vi "RC_STM_Client 1.vi"() -> ()   [LabVIEW 2019, in "RemoteControl.STM.lvclass"]
uses:
  RemoteControl.STM.lvclass
  RemoteControl/RemoteControl.lvclass
  <userlib>/_OpenG.lib/numeric/numeric.llb/Random Number Within Range - I32__ogtk.vi
  <userlib>/_OpenG.lib/error/error.llb/Filter Error Codes (Array)__ogtk.vi
  RemoteControl/Typedefs/RC Com Type--enum.ctl
panel:
  in  "Test RC Client":bool
  in  "milliseconds to wait":u32
  out "time (1 message) (ms)":u32
  out "startup time (ms)":u32
  out "messsages/s":dbl
  in  "remote port":u16=6341
  in  "address":string
  out "Data reponse":string
  out "Messages":i32
  in  "Stop":bool
  out "Command reponse":string
  out "Command":string
  out "meta data\n(available commands)":string
  out "error out":errorcluster
  # "CLIENT (API)"
  # "Connection info"
  # "Message Sent"
  # "Message Received"
  # "Metrics"
  # "1"
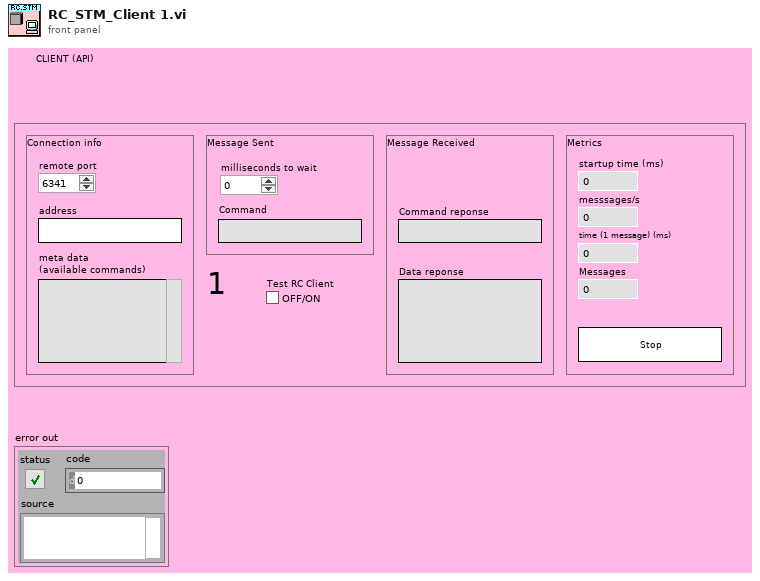
[diagram p1: front panel]
types:
  T1 = typedef "RemoteControl.lvclass/RC Com Type--enum.ctl" = enum16{"RC", "STM", "ZMQ"}
  T2 = typedef "NI STM.lvlib/MetaDataElement.ctl" = string
  T3 = cluster{"Command out":string, "Data out":variant, string}
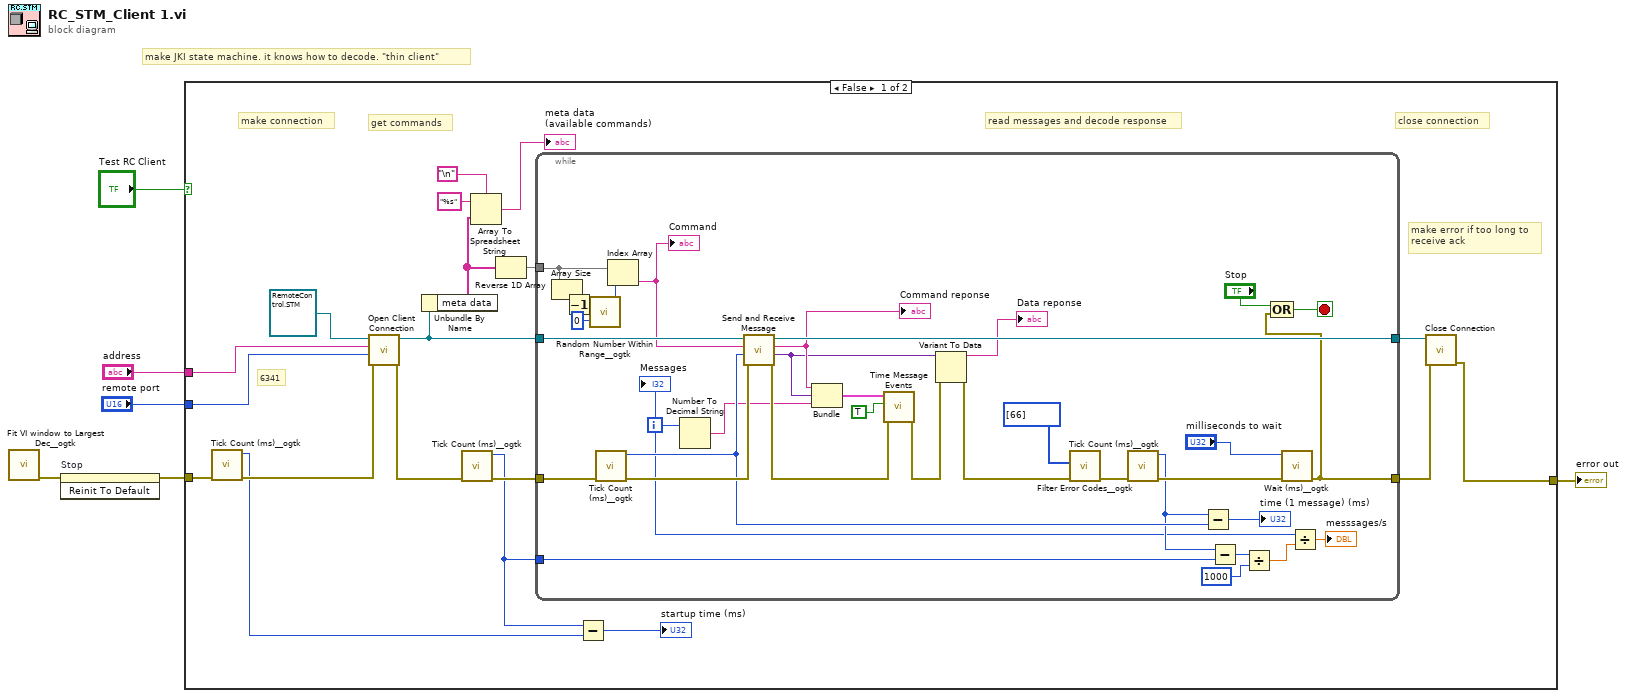
[diagram p0: block diagram]
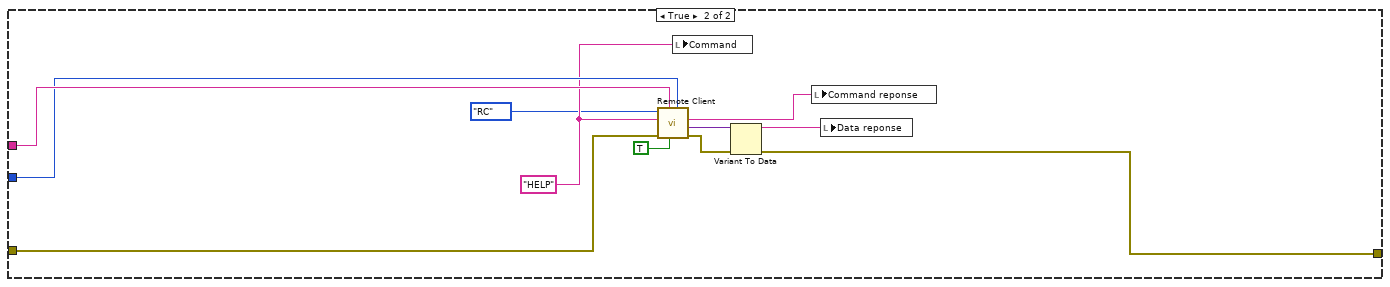
[diagram p2: hidden frame]
diagram:
  # "make JKI state machine. it knows how to decode. \"thin client\""
  n1 = call <userlib>:"Fit VI window to Largest Dec__ogtk.vi"() -> ("error out"=w2:errorcluster)  [unwired: 6 in, 1 out]
  n2 = invoke on="Stop" class="Bool" method="Reinit To Default"(error in=w2) -> (error out=w3:errorcluster)  [unwired: 2 in, 2 out]
  n3 = case shown="False" "Test RC Client" {
    tunnel: "remote port" -> [w11 w64]
    tunnel: "address" -> [w10 w65]
    tunnel: w3 -> [w9 w66]
    tunnel: [w8 w67] -> w1
    frame False {
      # "close connection"
      # "read messages and decode response"
      # "get commands"
      # "make connection"
      # "6341"
      # "make error if too long to\nreceive ack"
      n4 = call <userlib>:"Tick Count (ms)__ogtk.vi"("error in (no error)"=w9) -> ("error out"=w21:errorcluster, "millisecond timer value"=w17:u32)  [unwired: 9 in]
      n5 = call-dynamic "Open Client Connection.vi"("error in (no error)"=w21, "Port"=w11, "address"=w10, "RemoteControl.STM in"=refnum<class "RemoteControl.STM.lvclass"> refnum) -> ("error out"=w20:errorcluster, "RemoteControl.STM out"=w23:refnum<class "RemoteControl.STM.lvclass">)  [unwired: 6 in]
      n6 = Unbundle By Name(w23) -> ("meta data"=w16:T2[])
      n7 = call <userlib>:"Tick Count (ms)__ogtk.vi"("error in (no error)"=w20) -> ("error out"=w19:errorcluster, "millisecond timer value"=w12:u32)  [unwired: 9 in]
      n8 = Array To Spreadsheet String(delimiter (Tab)="\n", array=w16, 3:"%s" ("format string")) -> (spreadsheet string=→"meta data\n(available commands)":string)
      n9 = Reverse 1D Array(array=w16) -> (reversed array=w22:T2[])
      n10 = while {
        tunnel: [w37] -> w25
        tunnel: [w57] -> w24
        tunnel: w19 -> [w52]
        tunnel: w23 -> [w58]
        tunnel: w22 -> [w41]
        tunnel: w12 -> [w28]
        i -> [w27]
        stop <- w60 stop-if-true
        n11 = Array Size(array=w41) -> (size(s)=w42:i32)
        n12 = Decrement(x=w42) -> (x-1=w40:i32)
        n13 = call-poly <userlib>:"Random Number Within Range__ogtk.vi"("High"=w40, "Low"=0) -> ("Random Number"=w44:i32)  [unwired: 3 in]
        n14 = call <userlib>:"Tick Count (ms)__ogtk.vi"("error in (no error)"=w52) -> ("error out"=w51:errorcluster, "millisecond timer value"=w38:u32)  [unwired: 9 in]
        n15 = Index Array(array=w41, index=w44) -> (element=w53:T2)
        "Command" <- w53
        n16 = Number To Decimal String(number=w27) -> (decimal integer string=w26:string)  [unwired: 1 in]
        n17 = call-dynamic "Send and Receive Message.vi"("error in (no error)"=w51, "Data"=w38, "Command"=w53, "RemoteControl in"=w58) -> ("error out"=w39:errorcluster, "Data out"=w36:variant, "Command out"=w50:string, "RemoteControl out"=w57:refnum<class "RemoteControl.STM.lvclass">)  [unwired: 4 in]
        "Command reponse" <- w50
        n18 = Bundle("Command out"=w50, "Data out"=w36, w26) -> (w49:T3)  [unwired: 1 in]
        n19 = call "Time Message Events.vi"("error in (no error)"=w39, "Debug Mode"=TRUE, "Message in"=w49) -> ("error out"=w35:errorcluster)  [unwired: 6 in, 2 out]
        n20 = Variant To Data(error in=w35, Variant=w36) -> (data=→"Data reponse":string, error out=w34:errorcluster)  [unwired: 1 in]
        n21 = call-poly <userlib>:"Filter Error Codes__ogtk.vi"("Error In"=w34, "Error Codes to Filter"=i32[] [66]) -> ("Error Out"=w56:errorcluster)  [unwired: 7 in, 2 out]
        n22 = call <userlib>:"Tick Count (ms)__ogtk.vi"("error in (no error)"=w56) -> ("error out"=w47:errorcluster, "millisecond timer value"=w30:u32)  [unwired: 9 in]
        n23 = Subtract(x=w30, y=w38) -> (x-y=→"time (1 message) (ms)":u32)
        n24 = Subtract(x=w30, y=w28) -> (x-y=w29:u32)
        n25 = Divide(x=w29, y=u32 1000) -> (x/y=w55:dbl)
        n26 = call <userlib>:"Wait (ms)__ogtk.vi"("error in (no error)"=w47, "milliseconds to wait"="milliseconds to wait") -> ("error out"=w37:errorcluster)  [unwired: 8 in, 1 out]
        n27 = Compound Arithmetic op=OR("Stop", w37) -> (w60:bool)
        n28 = Divide(x=w27, y=w55) -> (x/y=→"messsages/s":dbl)
        "Messages" <- w27
      }
      n29 = Subtract(x=w12, y=w17) -> (x-y=→"startup time (ms)":u32)
      n30 = call-dynamic "Close Connection.vi"("error in (no error)"=w25, "RemoteControl.STM in"=w24) -> ("error out"=w8:errorcluster)  [unwired: 8 in, 1 out]
    }
    frame True {
      w63 = "HELP" ("Command")
      n31 = call "Remote Client.vi"("Port"=w64, "Wait for Response?"=TRUE, "address"=w65, "error in (no error)"=w66, "Command"=w63, "RC Type"=RC_Com_Type--enum."RC") -> ("error out"=w68:errorcluster, "Data out"=w71:variant, "Command out"=w70:string)  [unwired: 2 in, 1 out]
      n32 = local write "Command"(w63) -> ()
      n33 = Variant To Data(error in=w68, Variant=w71) -> (data=w69:string, error out=w67:errorcluster)  [unwired: 1 in]
      n34 = local write "Command reponse"(w70) -> ()
      n35 = local write "Data reponse"(w69) -> ()
    }
  }
  "error out" <- w1
